vi "Cluster Scrollbar Visible.vi"(8 "error in":errorcluster, 9 "Horizontal Scrollbar Visible":bool, 10 "Vertical Scrollbar Visible":bool, 11 "reference":refnum<vi>) -> (0 "error out":errorcluster)   [LabVIEW 2015]
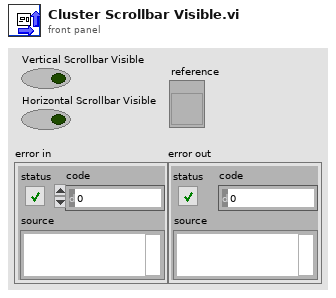
[diagram p1: front panel]
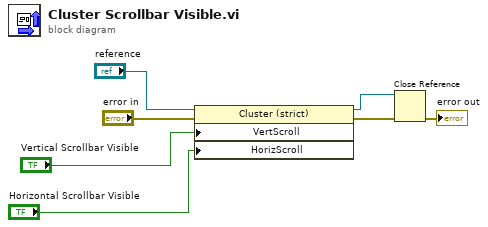
[diagram p0: block diagram]
diagram:
  n1 = property on="Property Node" class="Cluster (strict)"(reference="reference", error in="error in", "VertScroll"="Vertical Scrollbar Visible", "HorizScroll"="Horizontal Scrollbar Visible") -> (reference out=w3:refnum<vi>, error out=w4:errorcluster)
  n2 = Close Reference(reference=w3, error in (no error)=w4) -> (error out=→"error out":errorcluster)
